vi "playMacro.vi"(8 "error in (no error)":errorcluster, 10 "macro":string, 11 "VGS_RemoteControlClient in":refnum<class "VGS_RemoteControlClient.lvclass">) -> (0 "error out":errorcluster, 3 "VGS_RemoteControlClient out":refnum<class "VGS_RemoteControlClient.lvclass">)   [LabVIEW 2022 SP3, in "LV_VGS.lvlib" / "VGS_RemoteControlClient.lvclass"]
doc: "<B>Plays a recorded macro on the currently loaded VG project. </B>\n\nParameters\nhandle A valid remote handle. \nmacro The absolute path to a VG macro file (.vgc) is passed. \n\nEmit error ApplicationHasNoMacroSupportException if the current application instance has no macro support e.g. VGStudio or myVGL. \nEmit error RemoteControlServiceIsNotAvailableException if the remote control service doesn't run. \nEmit error GenericRemoteControlErrorException if an internal error occurs.\nEmit error InvalidRemoteHandleException if the remote handle is not valid. \n\nAttention\nThis method has been superceded by RemoteControlClient::runJob"
uses:
  VGS_RemoteControlClient.lvclass
  VGS_RemoteControlClient.lvclass/VGS_RemoteControlClient.ctl
  C:/Users/Andrey/Desktop/hajo/LV_VGS/vgs_project.dll
  vgs_project.dll
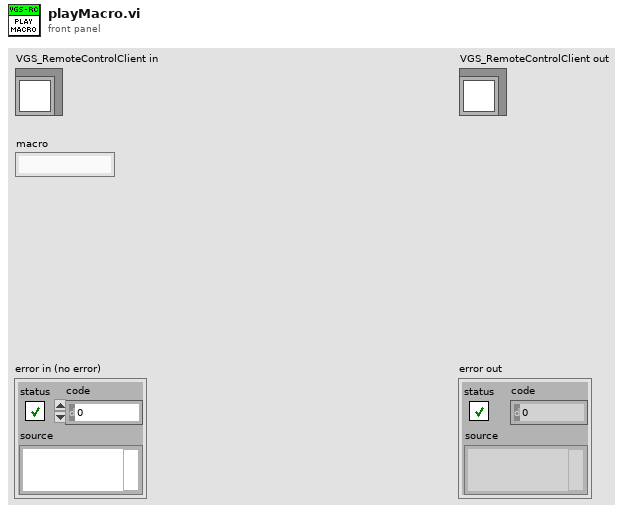
[diagram p1: front panel]
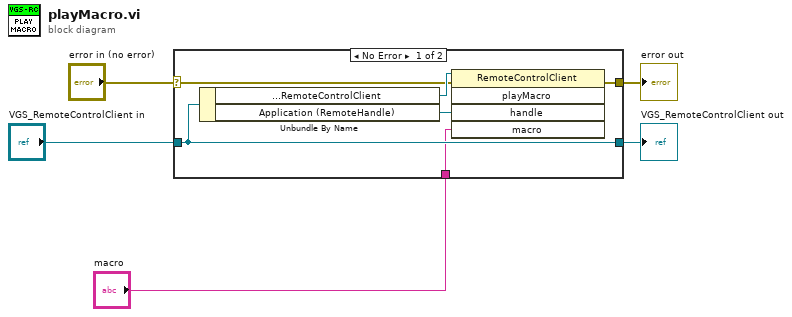
[diagram p0: block diagram]
diagram:
  n1 = case shown="No Error" "error in (no error)" {
    selector: "error in (no error)" -> [w8 w12]
    tunnel: [w7 w12] -> w4
    tunnel: [w11 w13] -> w2
    tunnel: "VGS_RemoteControlClient in" -> [w11 w13]
    tunnel: "macro" -> [w6 _]
    frame No Error {
      n2 = Unbundle By Name(w11) -> ("VGS.Project.Interop.RemoteControlClient"=w10:refnum<k24>, "Application (RemoteHandle)"=w9:refnum<k24>)
      n3 = invoke class="RemoteControlClient" method="playMacro"(reference=w10, error in=w8, "handle"=w9, "macro"=w6) -> (error out=w7:errorcluster)  [unwired: 1 in, 4 out]
    }
    frame Error {
    }
  }
  "error out" <- w4
  "VGS_RemoteControlClient out" <- w2
